vi "UpdateGraphRefPar.vi"(8 "error in (no error)":errorcluster caption="entrée d'erreur (pas d'erreur)", 9 "CurvIndex":i32, 10 "NewGraphIndex":i32, 11 "Interface en entrée":refnum<class "Interface.lvclass"> caption="DNL_LabVIEW Object in") -> (0 "error out":errorcluster caption="sortie d'erreur", 2 "CurvIndex Out":i32, 3 "Interface en sortie":refnum<class "Interface.lvclass"> caption="DNL_LabVIEW Object out")   [LabVIEW 2019, in "Interface.lvclass"]
uses:
  Interface.lvclass
  Interface.lvclass/Interface.ctl
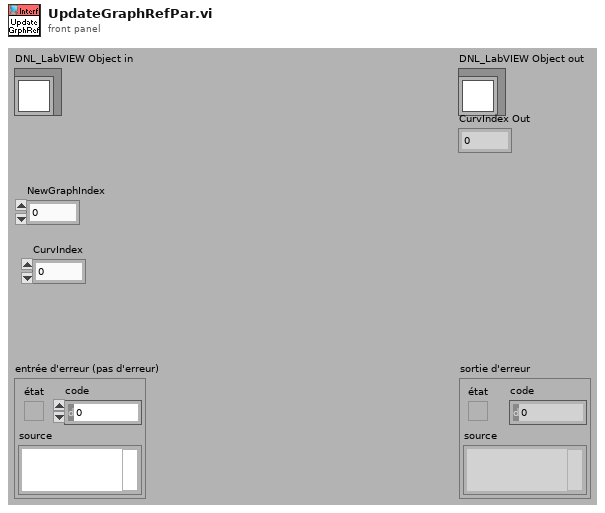
[diagram p1: front panel]
types:
  T1 = typedef "Interface.lvclass/CurveSetup.ctl" = cluster{"CurveName":string, "YParam":string, "XParam":string, "ZParam ":string, "GroupName":string, "LinWdth":u8, "PntCol":u32, "LinCol":u32, "LablFor":u8, "XScale":u32, "YScale":u32, "Interpol":u8, "DisplayName":string, "FillType":i16, "LineStyle":u8, "PntStyle":u8, "BarTyp":u8, "GraphIndex":i32, "Visible":bool, "XScaleName":string, "YScaleName":string, "XYGraph_Ref":refnum<vi>, "Data Only":bool, "DataQ Ref":refnum<queue>, "XParQ Ref":refnum<queue>, "XParamInd":i32, "ScanInd":i32}
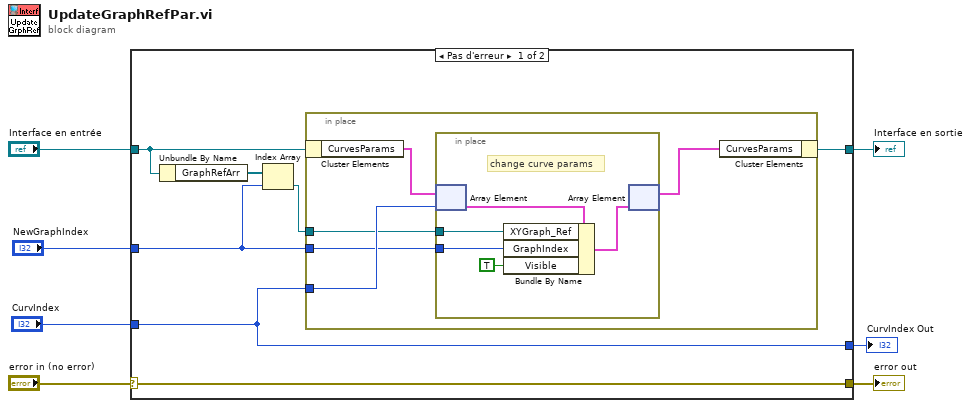
[diagram p0: block diagram]
diagram:
  n1 = case shown="Pas d'erreur" "error in (no error)" {
    selector: "error in (no error)" -> [w14 w27]
    tunnel: [w14 w27] -> w6
    tunnel: [w10 w26] -> w4
    tunnel: "Interface en entrée" -> [w13 w26]
    tunnel: "CurvIndex" -> [w9 w25]
    tunnel: "NewGraphIndex" -> [w8 _]
    tunnel: [w9 w25] -> w1
    frame No Error {
      n2 = Unbundle By Name(w13) -> ("GraphRefArr"=w12:refnum<vi>[])
      n3 = Index Array(array=w12, index=w8) -> (element=w11:refnum<vi>)
      n4 = in-place {
        in-place-border: w9 -> [w19]
        in-place-border: w11 -> [w18]
        in-place-border: w8 -> [w17]
        n5 = in-place-cluster #1(w13) -> ("CurvesParams"=w16:T1[])
        n6 = in-place {
          in-place-border: w18 -> [w23]
          in-place-border: w17 -> [w21]
          # "change curve params"
          n7 = in-place-array #2(w16, w19) -> (w22:T1)
          n8 = Bundle By Name(cluster=w22, "XYGraph_Ref"=w23, "GraphIndex"=w21, "Visible"=TRUE) -> (w24:T1)
          n9 = in-place-array #2(w24) -> (w15:T1[])  [unwired: 1 out]
        }
        n10 = in-place-cluster #1("CurvesParams"=w15) -> (w10:refnum<class "Interface.lvclass">)
      }
    }
    frame Error {
    }
  }
  "error out" <- w6
  "Interface en sortie" <- w4
  "CurvIndex Out" <- w1
